vi "Replace Array Subset (Value).vi"(5 "JSON Array":refnum<class "JSON Value.lvclass">, 7 "index":i32, 9 "new element/subarray":refnum<class "JSON Value.lvclass">, 11 "error in":errorcluster) -> (6 "output JSON Array":refnum<class "JSON Value.lvclass">, 15 "error out":errorcluster)   [LabVIEW 2016, in "JSON Value.lvclass"]
doc: "Replaces an element or subarray in an array at the point you specify in index."
uses:
  JSON Value.lvclass
  JSON Value.lvclass/JSON Value.ctl
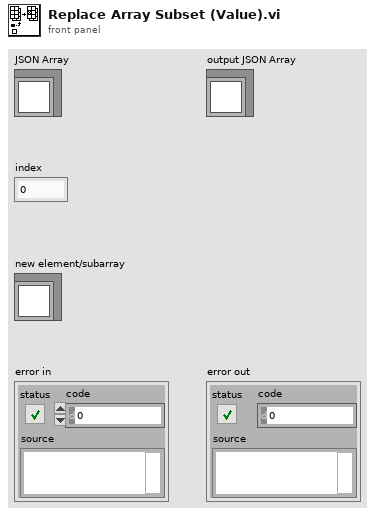
[diagram p1: front panel]
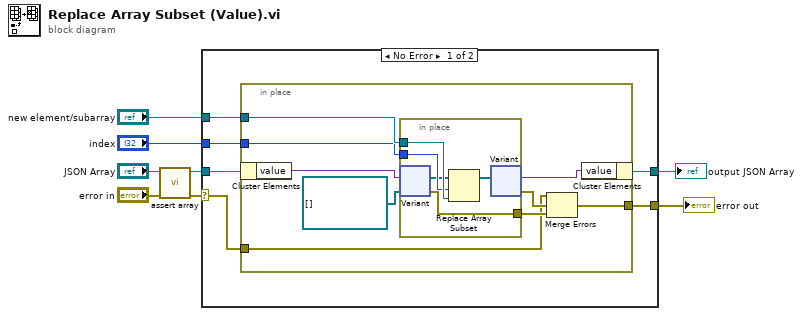
[diagram p0: block diagram]
diagram:
  n1 = call "assert array.vi"("error in (no error)"="error in", "JSON Value in"="JSON Array") -> ("error out"=w3:errorcluster, "JSON Value out"=w1:refnum<class "JSON Value.lvclass">)  [unwired: 8 in]
  n2 = case shown="No Error" w3 {
    selector: w3 -> [w9 w30]
    tunnel: w1 -> [w14 w29]
    tunnel: "new element/subarray" -> [w13 _]
    tunnel: "index" -> [w12 _]
    tunnel: [w11 w29] -> w6
    tunnel: [w10 w30] -> w5
    frame No Error {
      n3 = in-place {
        in-place-border: w13 -> [w23]
        in-place-border: w12 -> [w22]
        in-place-border: [w16] -> w10
        in-place-border: w9 -> [w15]
        n4 = in-place-cluster #1(w14) -> ("value"=w21:variant)
        n5 = in-place {
          in-place-border: w23 -> [w28]
          in-place-border: w22 -> [w27]
          in-place-border: [w24] -> w18
          n6 = in-place-variant #2(w21, refnum<class "JSON Value.lvclass">[] [] ("new element/subarray")) -> (w26:refnum<class "JSON Value.lvclass">[], w24:errorcluster)
          n7 = Replace Array Subset(array=w26, new element=w28, index=w27) -> (w25:refnum<class "JSON Value.lvclass">[])
          n8 = in-place-variant #2(w25) -> (w20:variant, w17:errorcluster)
        }
        n9 = Merge Errors(w15, w17, w18) -> (w16:errorcluster)
        n10 = in-place-cluster #1("value"=w20) -> (w11:refnum<class "JSON Value.lvclass">)
      }
    }
    frame Error {
    }
  }
  "output JSON Array" <- w6
  "error out" <- w5
